vi "filterStringsToString.vi"(11 "filterStrings":string[](array[string])) -> (3 "flatString":string)   [LabVIEW 2021]
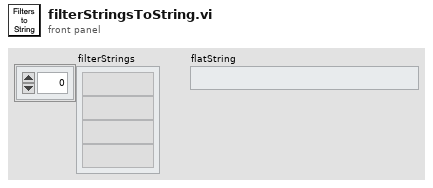
[diagram p1: front panel]
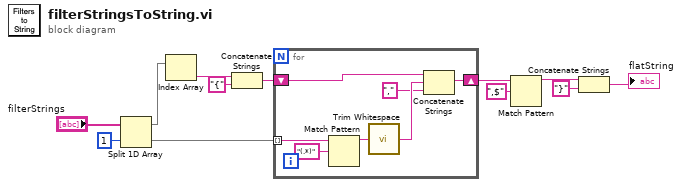
[diagram p0: block diagram]
diagram:
  n1 = Split 1D Array(array="filterStrings", index=1) -> (first subarray=w10:string[], second subarray=w11:string[])
  n2 = Index Array(array=w10) -> (element=w12:string)  [unwired: 1 in]
  n3 = Concatenate Strings(w12, "{" ("string")) -> (w7:string)
  n4 = for {
    shift-right: [w18] -> w3
    shift-left: w7 -> [w19]
    tunnel: w11 -> [w17] mode=indexing
    n5 = Match Pattern(string=w17, regular expression="(.*)") -> (before substring=w15:string)  [unwired: 1 in, 3 out]
    n6 = call <vilib>:"Trim Whitespace.vi"("string"=w15) -> ("trimmed string"=w14:string)  [unwired: 1 in]
    n7 = Concatenate Strings(w19, w14, "," ("string")) -> (w18:string)
  }
  n8 = Match Pattern(string=w3, regular expression=",$") -> (before substring=w1:string)  [unwired: 1 in, 3 out]
  n9 = Concatenate Strings(w1, "}" ("string")) -> (→"flatString":string)
